vi "Windows Test FDM Parse.vi"() -> ()   [LabVIEW 2010]
uses:
  FGNetFDM.ctl
  FlightGearState.ctl
  Flight Gear Data Custom Device.lvlib
panel:
  out "DBL Array":dbl[](array[numeric])
  out "Cluster":T1={"Version"={"version"=20, "pad"=0}, "Positions"={"Doubles"={"longitude"=0.0, "latitude"=0.0, "altitude"=0.0}, "Singles"={"agl"=0.0, "phi"=0.0, "theta"=0.0, "psi"=0.0, "alpha"=0.0, "beta"=0.0}}, "Velocities"={"phidot"=0.0, "thetadot"=0.0, "psidot"=0.0, "vcas"=0.0, "climb_rate"=0.0, "v_north"=0.0, "v_east"=0.0, "v_down"=0.0, "v_wind_body_north"=0.0, "v_wind_body_east"=0.0, "v_wind_body_down"=0.0}, "Accelerations"={"A_X_pilot"=0.0, "A_Y_pilot"=0.0, "A_Z_pilot"=0.0}, "Stall"={"stall_warning"=0.0, "slip_deg"=0.0}, "Engine Status"={"num_engines"=0, "eng_state"=[0, 0, 0, 0], "rpm"=[0.0, 0.0, 0.0, 0.0], "fuel_flow"=[0.0, 0.0, 0.0, 0.0], "fuel_px"=[0.0, 0.0, 0.0, 0.0], "egt"=[0.0, 0.0, 0.0, 0.0], "cht"=[0.0, 0.0, 0.0, 0.0], "mp_osi"=[0.0, 0.0, 0.0, 0.0], "tit"=[0.0, 0.0, 0.0, 0.0], "oil_temp"=[0.0, 0.0, 0.0, 0.0], "oil_px"=[0.0, 0.0, 0.0, 0.0]}, "Consumables"={"num_tanks"=0, "fuel_quantity"=[0.0, 0.0, 0.0, 0.0]}, "Gear Status"={"num_wheels"=0, "wow"=[0, 0, 0, 0], "gear_pos"=[0.0, 0.0, 0.0, 0.0], "gear_steer"=[0.0, 0.0, 0.0, 0.0], "gear_compression"=[0.0, 0.0, 0.0, 0.0]}, "Environment"={"curr_time"=0, "warp"=0, "visibility"=0.0}, "Control Surface Positions"={"elevator"=0.0, "elevator_trim_tab"=0.0, "left_flap"=0.0, "right_flap"=0.0, "left aileron"=0.0, "right_aileron"=0.0, "rudder"=0.0, "nose_wheel"=0.0, "speedbrake"=0.0, "spoilers"=0.0}}
  out "error out":errorcluster
  in  "stop":bool
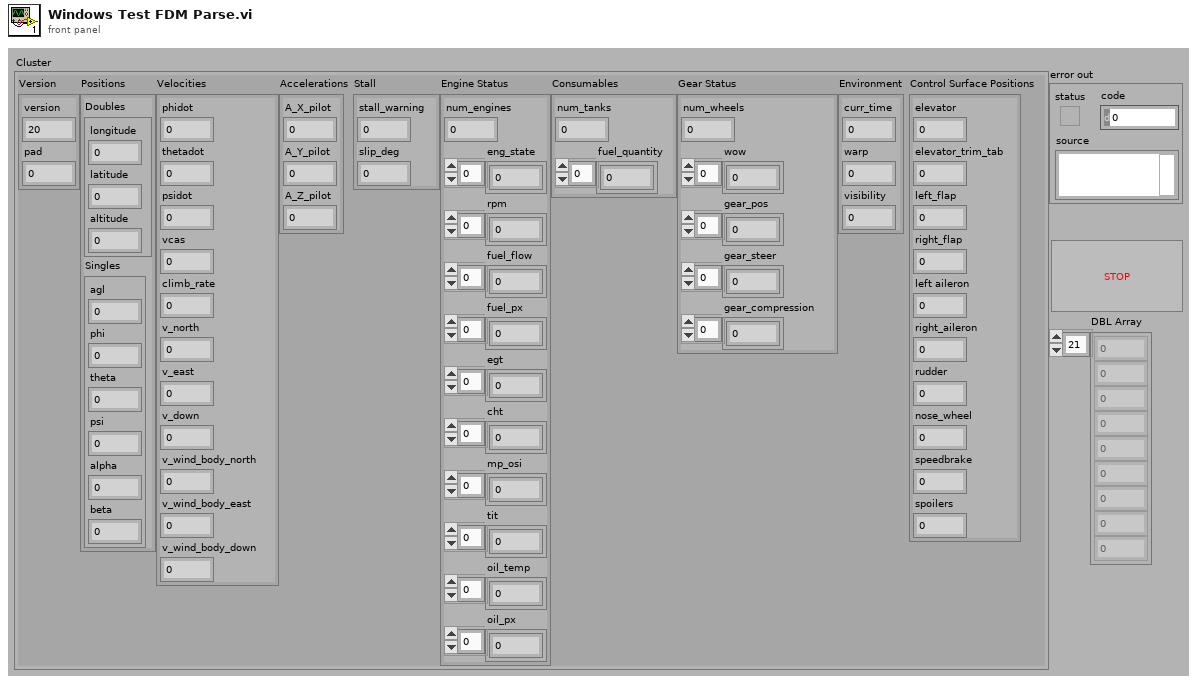
[diagram p1: front panel]
types:
  T1 = typedef "Flight Gear Data Custom Device.lvlib/FGNetFDM.ctl" = cluster{"Version":cluster{"version":u32, "pad":u32}, "Positions":cluster{"Doubles":cluster{"longitude":dbl, "latitude":dbl, "altitude":dbl}, "Singles":cluster{"agl":sgl, "phi":sgl, "theta":sgl, "psi":sgl, "alpha":sgl, "beta":sgl}}, "Velocities":cluster{"phidot":sgl, "thetadot":sgl, "psidot":sgl, "vcas":sgl, "climb_rate":sgl, "v_north":sgl, "v_east":sgl, "v_down":sgl, "v_wind_body_north":sgl, "v_wind_body_east":sgl, "v_wind_body_down":sgl}, "Accelerations":cluster{"A_X_pilot":sgl, "A_Y_pilot":sgl, "A_Z_pilot":sgl}, "Stall":cluster{"stall_warning":sgl, "slip_deg":sgl}, "Engine Status":cluster{"num_engines":u32, "eng_state":u32[], "rpm":sgl[], "fuel_flow":sgl[], "fuel_px":sgl[], "egt":sgl[], "cht":sgl[], "mp_osi":sgl[], "tit":sgl[], "oil_temp":sgl[], "oil_px":sgl[]}, "Consumables":cluster{"num_tanks":u32, "fuel_quantity":sgl[]}, "Gear Status":cluster{"num_wheels":u32, "wow":u32[], "gear_pos":sgl[], "gear_steer":sgl[], "gear_compression":sgl[]}, "Environment":cluster{"curr_time":u32, "warp":i32, "visibility":sgl}, "Control Surface Positions":cluster{"elevator":sgl, "elevator_trim_tab":sgl, "left_flap":sgl, "right_flap":sgl, "left aileron":sgl, "right_aileron":sgl, "rudder":sgl, "nose_wheel":sgl, "speedbrake":sgl, "spoilers":sgl}}
  T2 = typedef "Flight Gear Data Custom Device.lvlib/FlightGearState.ctl" = enum16{"Initialize", "Read", "Write", "Close"}
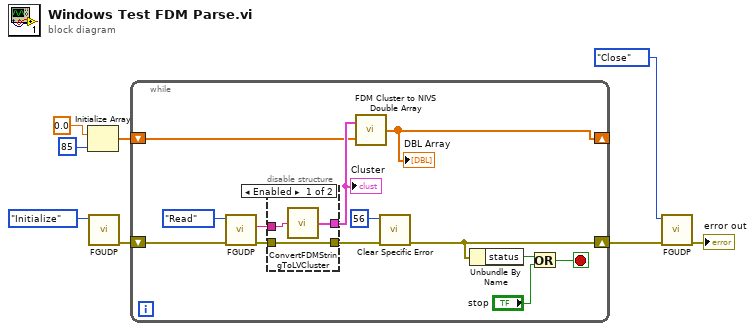
[diagram p0: block diagram]
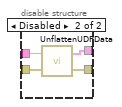
[diagram p2: hidden frame]
diagram:
  n1 = Initialize Array(0.0 ("element"), 85 ("dimension size")) -> (w3:dbl[])
  n2 = call "FGUDP.vi"("UDP State"=FlightGearState."Initialize") -> ("error out"=w8:errorcluster)  [unwired: 9 in, 1 out]
  n3 = while {
    shift-right: [w15] -> w7
    shift-left: w8 -> [w20]
    shift-right: [w11] -> _
    shift-left: w3 -> [w12]
    stop <- w19 stop-if-true
    n4 = call "FGUDP.vi"("Error In"=w20, "UDP State"=FlightGearState."Read") -> ("error out"=w10:errorcluster, "Data String Out"=w14:string)  [unwired: 8 in]
    n5 = disable-structure shown="Enabled" {
      disable-tunnel: w14 -> [w24 w28]
      disable-tunnel: [w23 w27] -> w13
      disable-tunnel: w10 -> [w22 w26]
      disable-tunnel: [w22 w25] -> w9
      frame Enabled {
        n6 = call "ConvertFDMStringToLVCluster.vi"("FGNetFDM"=w24) -> ("Cluster"=w23:T1)
      }
      frame Disabled {
        n7 = call "UnflattenUDPData.vi"("error in (no error)"=w26, "FGNetFDM"=w28) -> ("error out"=w25:errorcluster, "Cluster"=w27:T1)
      }
    }
    "Cluster" <- w13
    n8 = call "FDM Cluster to NIVS Double Array.vi"("Buffer In"=w12, "Cluster"=w13) -> ("DBL Array"=w11:dbl[])
    "DBL Array" <- w11
    n9 = call "Clear Specific Error.vi"("error in (no error)"=w9, "code"=56) -> ("error out"=w15:errorcluster)  [unwired: 9 in]
    n10 = Unbundle By Name(w15) -> ("status"=w18:bool)
    n11 = Or(x=w18, y="stop") -> (x .or. y?=w19:bool)
  }
  n12 = call "FGUDP.vi"("Error In"=w7, "UDP State"=FlightGearState."Close") -> ("error out"=→"error out":errorcluster)  [unwired: 8 in, 1 out]
